vi "Open and minimize VI by path.vi"(0 "LV DEV.lvclass":refnum<class "LV DEV.lvclass">, 5 "Vi Path":path, 11 "Error in":errorcluster) -> (4 "LV DEV.lvclass":refnum<class "LV DEV.lvclass">, 15 "Error Out":errorcluster)   [LabVIEW 2016, in "LV DEV.lvclass"]
doc: "Get reference of given VI."
uses:
  LV DEV.lvclass
  D:/Navin Workspace/MDI/source code/Document/LV Doc/LV Doc.lvclass
  LV DEV.lvclass/LV DEV.ctl
  LV Doc.lvclass/LV Doc.ctl
  property/Write application reference.vi
  property/Write VI Reference.vi
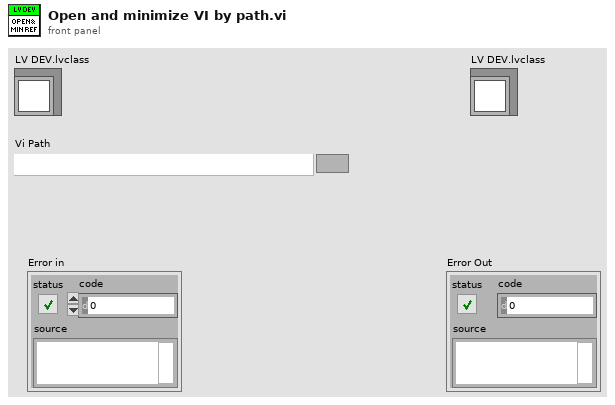
[diagram p1: front panel]
types:
  T1 = enum32{"Invalid", "Standard", "Closed", "Hidden", "Minimized", "Maximized"}
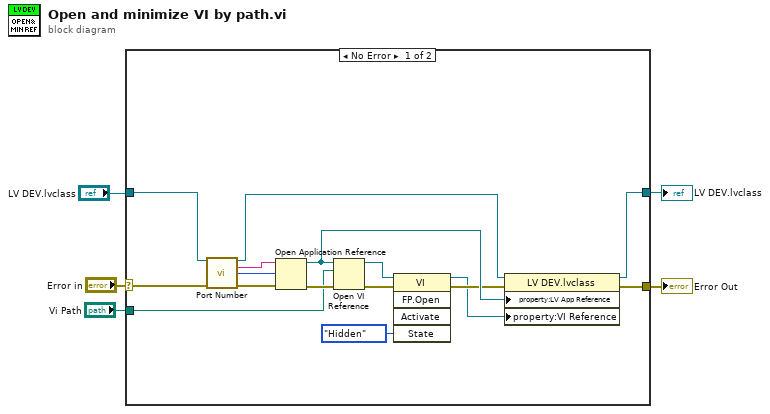
[diagram p0: block diagram]
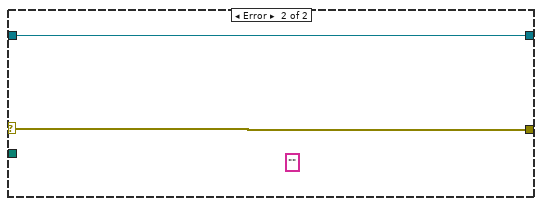
[diagram p2: hidden frame]
diagram:
  n1 = case shown="No Error" "Error in" {
    selector: "Error in" -> [w17 w23]
    tunnel: [w9 w23] -> w4
    tunnel: "Vi Path" -> [w12 _]
    tunnel: "LV DEV.lvclass" -> [w16 w22]
    tunnel: [w8 w22] -> w1
    frame No Error {
      n2 = call "Port Number.vi"("LV DEV.lvclass"=w16, "Error In"=w17) -> ("LV DEV.lvclass"=w11:refnum<class "LV DEV.lvclass">, "Machine name"=w14:string, "Port Number"=w13:u16, "error Out"=w15:errorcluster)  [unwired: 10 in]
      n3 = Open Application Reference(8:w15, 10:w13, 11:w14) -> (0:w19:errorcluster, 3:w10:refnum<vi>)  [unwired: 1 in]
      n4 = Open VI Reference(application reference (local)=w10, vi path=w12, error in (no error)=w19) -> (vi reference=w20:refnum<vi>, error out=w21:errorcluster)  [unwired: 3 in]
      n5 = invoke class="VI" method="FP.Open"(reference=w20, error in=w21, "State"=T1."Hidden") -> (reference out=w6:refnum<vi>, error out=w7:errorcluster)  [unwired: 2 in, 3 out]
      n6 = property class="LV DEV.lvclass"(reference=w11, error in=w7, "property:LV App Reference"=w10, "property:VI Reference"=w6) -> (reference out=w8:refnum<class "LV DEV.lvclass">, error out=w9:errorcluster)
    }
    frame Error {
      (unwired) "" ("Front Panel.Title")
    }
  }
  "Error Out" <- w4
  "LV DEV.lvclass" <- w1
